vi "getAllDevices.vi"(8 "error in (no error)":errorcluster, 11 "deviceDataBase in":refnum<class "deviceDataBase.lvclass">) -> (0 "error out":errorcluster, 2 "deviceArray.lvclass":refnum<class "DeviceArray.lvclass">, 3 "deviceDataBase out":refnum<class "deviceDataBase.lvclass">)   [LabVIEW 2009, in "Tools.lvlib" / "DatabaseHelpers.lvlib" / "deviceDataBase.lvclass"]
uses:
  deviceDataBase.lvclass
  Database Objects/DeviceArray/DeviceArray.lvclass
  deviceDataBase.lvclass/deviceDataBase.ctl
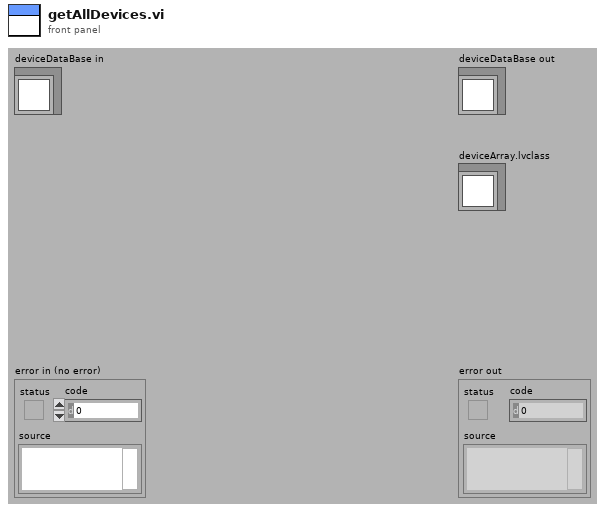
[diagram p1: front panel]
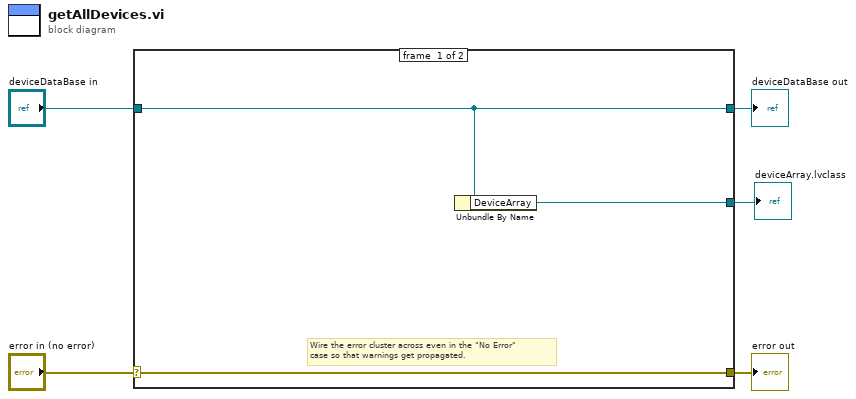
[diagram p0: block diagram]
diagram:
  n1 = case shown="No Error" "error in (no error)" {
    selector: "error in (no error)" -> [w8 w10]
    tunnel: [w8 w10] -> w4
    tunnel: [w7 w9] -> w2
    tunnel: "deviceDataBase in" -> [w7 w9]
    tunnel: [w6 _] -> w1
    frame #0 {
      # "Wire the error cluster across even in the \"No Error\"\ncase so that warnings get propagated."
      n2 = Unbundle By Name(w7) -> ("DeviceArray"=w6:refnum<class "DeviceArray.lvclass">)
    }
    frame #1 {
    }
  }
  "error out" <- w4
  "deviceDataBase out" <- w2
  "deviceArray.lvclass" <- w1
